vi "Remove Signals.vi"(8 "error in (no error)":errorcluster, 9 "Signal Array":T1[](array[typedef]), 10 "Action":T2, 11 "Custom Device reference in":refnum<k24>) -> (0 "error out":errorcluster, 3 "Custom Device reference out":refnum<k24>)   [LabVIEW 2013, in "J1939 System Definition API Support.lvlib"]
uses:
  J1939 System Definition API Support.lvlib
  NationalInstruments.VeriStand.SystemDefinitionAPI
  Types/Remove Frame Action.ctl
  Types/Remove Item - Frame Cluster.ctl
  Shared/SubVIs/Constants.vi
  <vilib>/NI Veristand/Custom Device Tools/Custom Device Utility Library/NI VeriStand - Search for All Items by GUID.vi
  <vilib>/NI Veristand/Custom Device Tools/Custom Device Utility Library/NI VeriStand - Search for Item by Name.vi
  <vilib>/NI Veristand/Custom Device Tools/Custom Device Utility Library/Custom Device Utility Library.lvlib
  <vilib>/NI Veristand/Custom Device API/Custom Device API.lvlib
  Shared/J1939 Addon Shared.lvlib
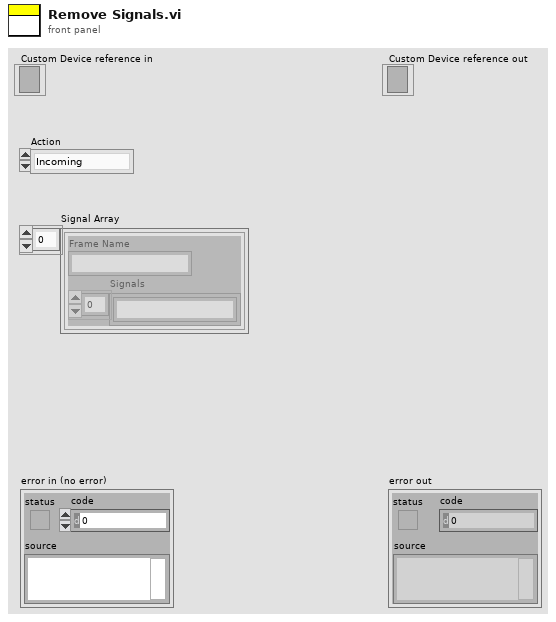
[diagram p1: front panel]
types:
  T1 = typedef "J1939 System Definition API Support.lvlib/Remove Item - Frame Cluster.ctl" = cluster{"Frame Name":string, "Signals":string[]}
  T2 = typedef "J1939 System Definition API Support.lvlib/Remove Frame Action.ctl" = enum16{"Incoming", "Outgoing"}
  T3 = typedef "Custom Device API.lvlib/Custom Device Item Ref.ctl" = u64
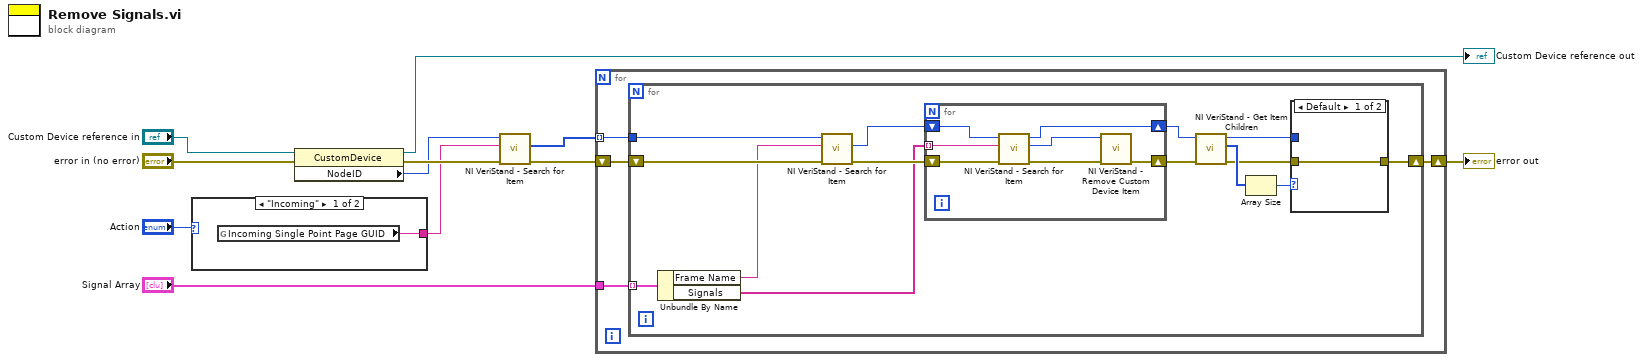
[diagram p0: block diagram]
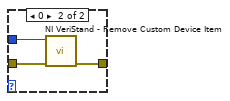
[diagram p2: hidden frame]
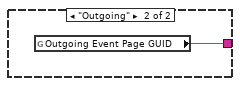
[diagram p3: hidden frame]
diagram:
  n1 = case shown="\"Incoming\"" "Action" {
    tunnel: [w12 w13] -> w7
    frame "Incoming" {
      n2 = global read "Constants.vi" "Incoming Single Point Page GUID"() -> (w12:string)
    }
    frame "Outgoing" {
      n3 = global read "Constants.vi" "Outgoing Event Page GUID"() -> (w13:string)
    }
  }
  n4 = property class="CustomDevice"(reference="Custom Device reference in", error in="error in (no error)") -> (reference out=→"Custom Device reference out":refnum<k24>, error out=w8:errorcluster, "NodeID"=w6:u64)
  n5 = call-poly <vilib>:"NI VeriStand - Search for Item.vi"("error in"=w8, "Item GUID"=w7, "Section Ref in"=w6) -> ("error out"=w4:errorcluster, "Item Refs"=w5:T3[])  [unwired: 5 in, 2 out]
  n6 = for {
    tunnel: w5 -> [w17] mode=indexing
    tunnel: "Signal Array" -> [w14]
    shift-right: [w15] -> w3
    shift-left: w4 -> [w16]
    n7 = for {
      tunnel: w17 -> [w31]
      tunnel: w14 -> [w28] mode=indexing
      shift-right: [w21] -> w15
      shift-left: w16 -> [w30]
      n8 = Unbundle By Name(w28) -> ("Frame Name"=w27:string, "Signals"=w26:string[])
      n9 = call-poly <vilib>:"NI VeriStand - Search for Item.vi"("error in"=w30, "Item Name"=w27, "Section Ref in"=w31) -> ("error out"=w29:errorcluster, "Item Ref"=w18:T3)  [unwired: 5 in, 2 out]
      n10 = for {
        shift-right: [w42] -> w24
        shift-left: w29 -> [w41]
        tunnel: w26 -> [w38] mode=indexing
        shift-right: [w36] -> w25
        shift-left: w18 -> [w39]
        n11 = call-poly <vilib>:"NI VeriStand - Search for Item.vi"("error in"=w41, "Item Name"=w38, "Section Ref in"=w39) -> ("error out"=w40:errorcluster, "Item Ref"=w37:T3, "Section Ref out"=w36:T3)  [unwired: 5 in, 1 out]
        n12 = call <vilib>:"NI VeriStand - Remove Custom Device Item.vi"("error in (no error)"=w40, "Item Ref in"=w37) -> ("error out"=w42:errorcluster)  [unwired: 8 in, 1 out]
      }
      n13 = call <vilib>:"NI VeriStand - Get Item Children.vi"("error in (no error)"=w24, "Item Ref in"=w25) -> ("error out"=w22:errorcluster, "Child Refs"=w23:T3[], "Item Ref out"=w19:T3)  [unwired: 6 in, 1 out]
      n14 = Array Size(array=w23) -> (size(s)=w20:i32)
      n15 = case shown="Default" w20 {
        tunnel: w22 -> [w32 w35]
        tunnel: [w32 w34] -> w21
        tunnel: w19 -> [_ w33]
        frame Default {
        }
        frame 0 {
          n16 = call <vilib>:"NI VeriStand - Remove Custom Device Item.vi"("error in (no error)"=w35, "Item Ref in"=w33) -> ("error out"=w34:errorcluster)  [unwired: 8 in, 1 out]
        }
      }
    }
  }
  "error out" <- w3
